vi "Manual Override.vi"(5 "Enable":bool, 7 "Override mode":T2=enum."STOP", 8 "Pivot Position Select":T1, 9 "Position Data":dbl, 10 "Percent Out Data":dbl, 11 "Auto CMD":T3) -> (3 "OverRide Command Out":T3)   [LabVIEW 2023, in "Pivot FX_ACT.lvlib"]
uses:
  Pivot FX_ACT.lvlib
  ENUM_CMD_Mode Select.ctl
  Cluster_CMD_ACT_Data.ctl
  Shared Code/TypeDefs/ENUM_Pivot Arm Position Select.ctl
  TRASH/xxxENUM_Override_Select.ctl
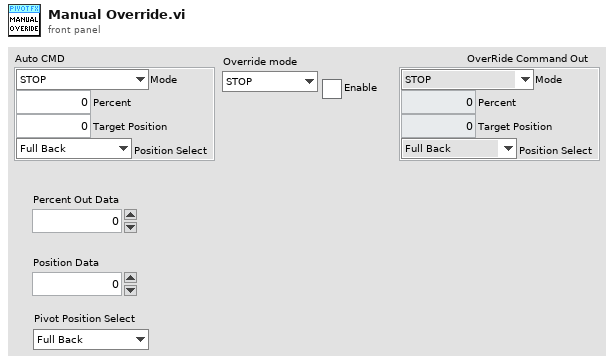
[diagram p1: front panel]
types:
  T1 = typedef "ENUM_Pivot Arm Position Select.ctl" = enum16{"Full Back", "Full Forward", "Amp Score", "Pivot Arm Load", "Vertical", "Trap Score"}
  T2 = typedef "xxxENUM_Override_Select.ctl" = enum16{"Teleop-Auto", "Percent Output", "Position Value", "Position Select", "STOP"}
  T3 = typedef "Pivot FX_ACT.lvlib/Cluster_CMD_ACT_Data.ctl" = cluster{"Mode":T4, "Percent":dbl, "Target Position":dbl, "Position Select":T1}
  T4 = typedef "Pivot FX_ACT.lvlib/ENUM_CMD_Mode Select.ctl" = enum16{"STOP", "PercentOut", "Positon Value", "Position Select"}
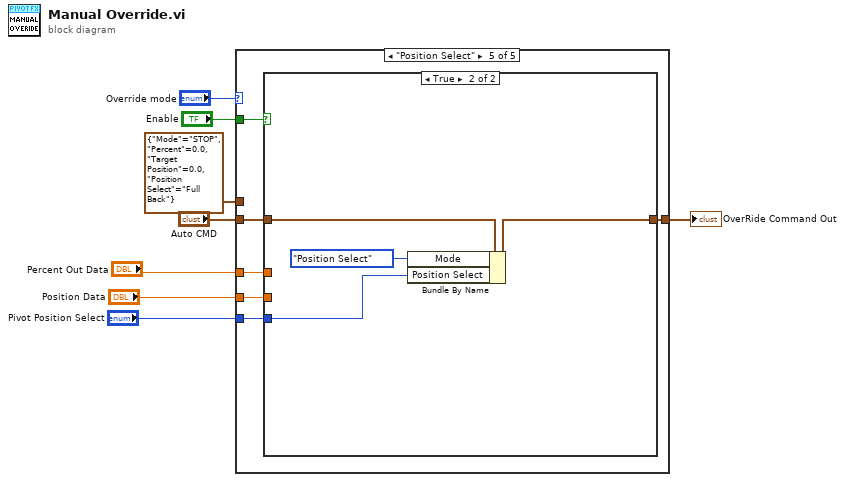
[diagram p0: block diagram]
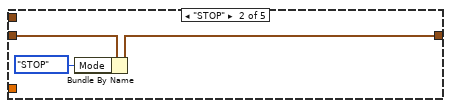
[diagram p3: hidden frame]
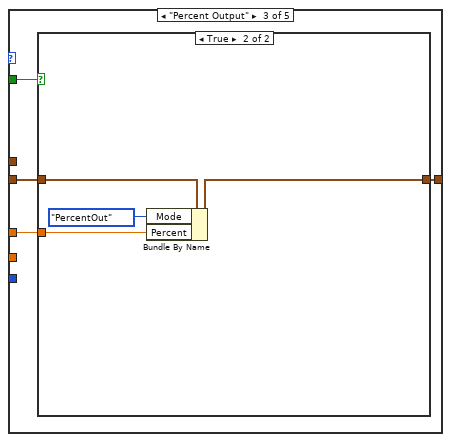
[diagram p4: hidden frame]
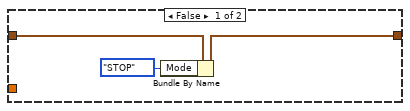
[diagram p5: hidden frame]
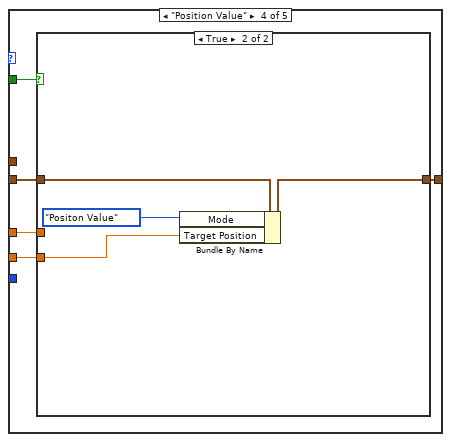
[diagram p6: hidden frame]
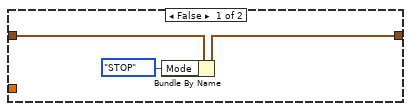
[diagram p7: hidden frame]
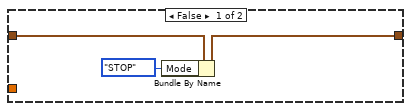
[diagram p8: hidden frame]
diagram:
  n1 = case shown="\"Position Select\"" "Override mode" {
    tunnel: [w9 w10 w15 w27 w40] -> w8
    tunnel: "Auto CMD" -> [w9 w11 w16 w28 w41]
    tunnel: T3 {"Mode"=enum."STOP", "Percent"=0.0, "Target Position"=0.0, "Position Select"=enum."Full Back"} ("OverRide Command Out") -> [_ _ _ _ _]
    tunnel: "Enable" -> [_ _ w14 w26 w39]
    tunnel: "Percent Out Data" -> [_ _ w13 w25 w38]
    tunnel: "Position Data" -> [_ _ _ w24 w37]
    tunnel: "Pivot Position Select" -> [_ _ _ _ w36]
    frame "Teleop-Auto" {
    }
    frame "STOP" {
      n2 = Bundle By Name(cluster=w11, "Mode"=ENUM_CMD_Mode_Select."STOP") -> (w10:T3)
    }
    frame "Percent Output" {
      n3 = case shown="True" w14 {
        tunnel: w16 -> [w18 w23]
        tunnel: [w17 w21] -> w15
        tunnel: w13 -> [_ w20]
        frame False {
          n4 = Bundle By Name(cluster=w18, "Mode"=ENUM_CMD_Mode_Select."STOP") -> (w17:T3)
        }
        frame True {
          n5 = Bundle By Name(cluster=w23, "Mode"=ENUM_CMD_Mode_Select."PercentOut", "Percent"=w20) -> (w21:T3)
        }
      }
    }
    frame "Position Value" {
      n6 = case shown="True" w26 {
        tunnel: w28 -> [w30 w35]
        tunnel: [w29 w33] -> w27
        tunnel: w25 -> [_ _]
        tunnel: w24 -> [_ w32]
        frame False {
          n7 = Bundle By Name(cluster=w30, "Mode"=ENUM_CMD_Mode_Select."STOP") -> (w29:T3)
        }
        frame True {
          n8 = Bundle By Name(cluster=w35, "Mode"=ENUM_CMD_Mode_Select."Positon Value", "Target Position"=w32) -> (w33:T3)
        }
      }
    }
    frame "Position Select" {
      n9 = case shown="True" w39 {
        tunnel: w41 -> [w43 w48]
        tunnel: [w42 w46] -> w40
        tunnel: w38 -> [_ _]
        tunnel: w37 -> [_ _]
        tunnel: w36 -> [_ w45]
        frame False {
          n10 = Bundle By Name(cluster=w43, "Mode"=ENUM_CMD_Mode_Select."STOP") -> (w42:T3)
        }
        frame True {
          n11 = Bundle By Name(cluster=w48, "Mode"=ENUM_CMD_Mode_Select."Position Select", "Position Select"=w45) -> (w46:T3)
        }
      }
    }
  }
  "OverRide Command Out" <- w8
